vi "Untitled 2.vi"() -> ()   [LabVIEW 2019]
panel:
  out "return value":string
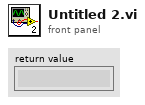
[diagram p1: front panel]
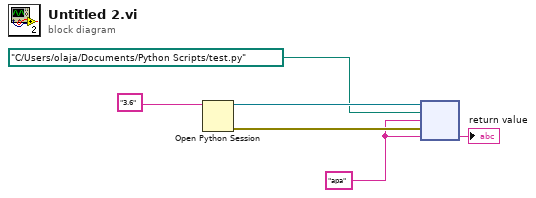
[diagram p0: block diagram]
diagram:
  w2 = "apa" ("function name")
  n1 = Open Python Session(python version="3.6" ("function name")) -> (session out=w6:refnum<k35>, error out=w3:errorcluster)  [unwired: 2 in]
  n2 = node(w6, path "C:/Users/olaja/Documents/Python Scripts/test.py" ("module path"), w2, w3, w2) -> (→"return value":string)  [unwired: 4 out]
